vi "PRAT Find Draw Index.vi"(8 "Error In":errorcluster, 9 "Finish Draw Count":i32[](array[numeric]), 10 "Start Draw Count":i32[](array[numeric]), 11 "Draw Count In":i32) -> (0 "Error Out":errorcluster, 3 "index of element":i32, 5 "Draw Count Out":i32)   [LabVIEW 2020]
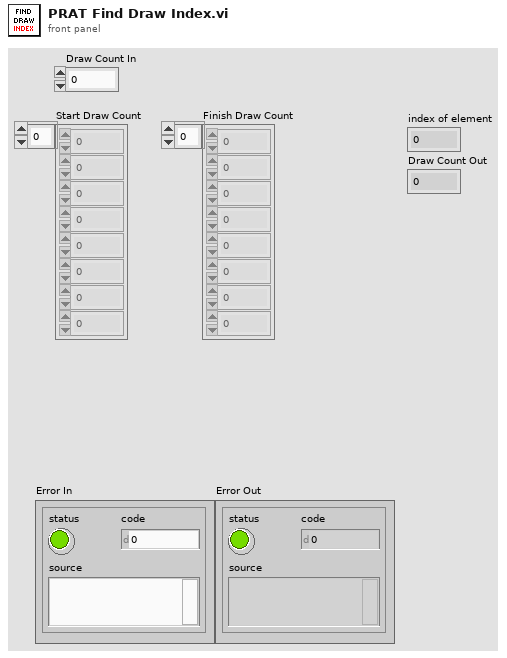
[diagram p1: front panel]
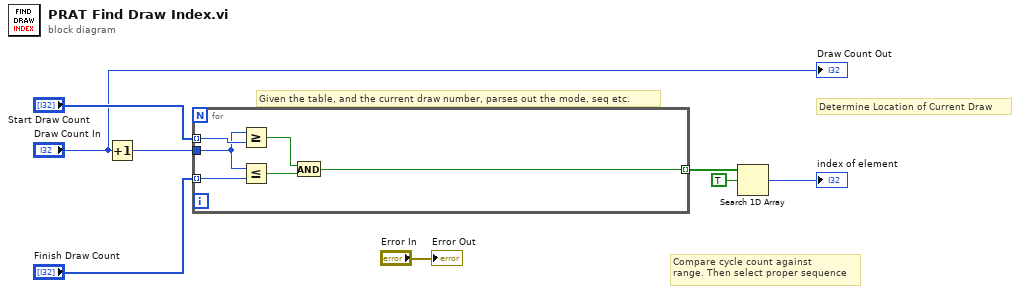
[diagram p0: block diagram]
diagram:
  # "Compare cycle count against\nrange. Then select proper sequence"
  # "Determine Location of Current Draw"
  # "Given the table, and the current draw number, parses out the mode, seq etc."
  n1 = Increment(x="Draw Count In") -> (x+1=w2:i32)
  n2 = for {
    tunnel: "Start Draw Count" -> [w14] mode=indexing
    tunnel: "Finish Draw Count" -> [w12] mode=indexing
    tunnel: w2 -> [w13]
    tunnel: [w9] -> w6 mode=indexing
    n3 = Greater Or Equal?(x=w13, y=w14) -> (x >= y?=w11:bool)
    n4 = Less Or Equal?(x=w13, y=w12) -> (x <= y?=w10:bool)
    n5 = And(x=w11, y=w10) -> (x .and. y?=w9:bool)
  }
  n6 = Search 1D Array(1D array=w6, element=TRUE) -> (index of element=→"index of element":i32)  [unwired: 1 in]
  "Error Out" <- "Error In"
  "Draw Count Out" <- "Draw Count In"
